vi "Write Objects.vi"(8 "error in":errorcluster, 10 "Objects":T1[](array[typedef]) {"Object ID" format="%x"}, 11 "device data model in":refnum<class "Device Data Model.lvclass">) -> (0 "error out":errorcluster, 3 "device data model out":refnum<class "Device Data Model.lvclass">)   [LabVIEW 2012, in "Device Data Model.lvclass"]
doc: "Writes objects to the device model. This function overwrites existing objects."
uses:
  Device Data Model.lvclass
  Identification Parameters.ctl
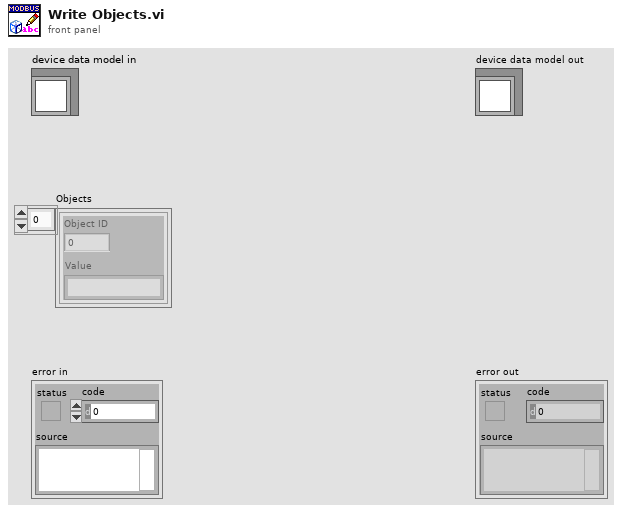
[diagram p1: front panel]
types:
  T1 = typedef "Device Data Model.lvclass/Identification Parameters.ctl" = cluster{"Object ID":u8, "Value":string}
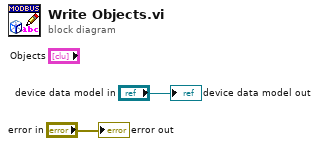
[diagram p0: block diagram]
diagram:
  "error out" <- "error in"
  "device data model out" <- "device data model in"
